vi "Post Build Script (auto build).vi"(7 "Project File Path":path, 8 "Package Source Folder":path, 9 "Package Version (Major.Minor.Fix.Build)":string, 10 "Product Name":string, 11 "Output Package File Path":path) -> (0 "error out":errorcluster)   [LabVIEW 2019, in "PostBuildSupport.lvclass"]
doc: "This VI will execute the build specs inside the project in order to build an Application and Installer. It will then create a single self-extracting installer file. It is meant to be placed inside \"Post-Build Custom Action.vi\" that is called post VIPM package build."
uses:
  PostBuildSupport.lvclass
  PostBuildSupport.lvclass/PostBuildSupport.ctl
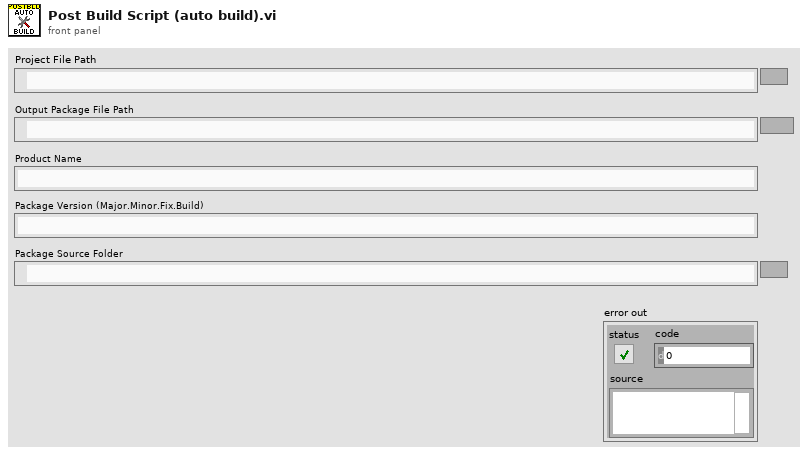
[diagram p1: front panel]
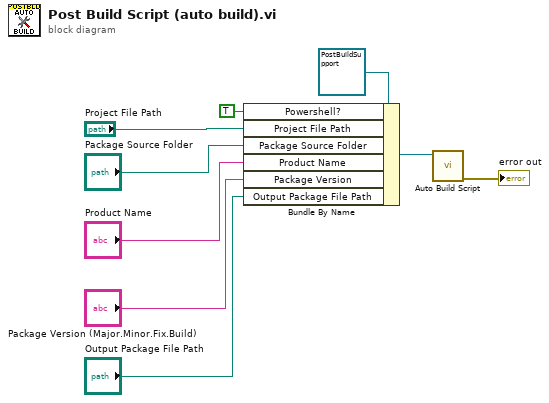
[diagram p0: block diagram]
diagram:
  n1 = Bundle By Name(cluster=refnum<class "PostBuildSupport.lvclass"> refnum ("PostBuildSupport in"), "Powershell?"=TRUE, "Project File Path"="Project File Path", "Package Source Folder"="Package Source Folder", "Product Name"="Product Name", "Package Version"="Package Version (Major.Minor.Fix.Build)", "Output Package File Path"="Output Package File Path") -> (w4:refnum<class "PostBuildSupport.lvclass">)
  n2 = call "Auto Build Script.vi"("PostBuildSupport"=w4) -> ("error out"=→"error out":errorcluster)  [unwired: 10 in]
